vi "GetCtrlData.vi"(8 "error in (no error)":errorcluster, 11 "Panel in":refnum<vi>) -> (0 "error out":errorcluster, 2 "Indicators":string[][](array[string]), 3 "Controls":string[][](array[string]))   [LabVIEW 2016, in "update vi properties.lvlib"]
uses:
  update vi properties.lvlib
panel:
  # "Connector Pane"
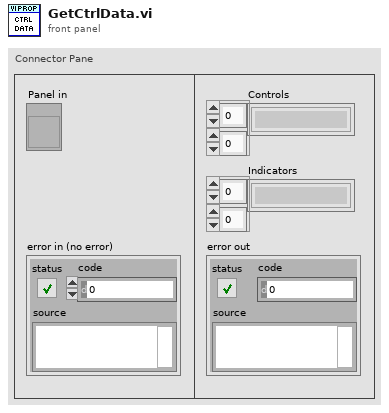
[diagram p1: front panel]
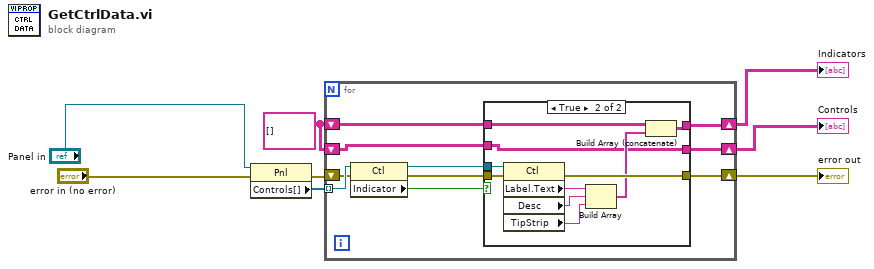
[diagram p0: block diagram]
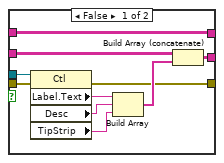
[diagram p2: hidden frame]
diagram:
  w8 = string[][] []
  n1 = property class="Pnl"(reference="Panel in", error in="error in (no error)") -> (error out=w7:errorcluster, "Controls[]"=w6:refnum<vi>[])  [unwired: 1 out]
  n2 = for {
    tunnel: w6 -> [w18] mode=indexing
    shift-right: [w13] -> w5
    shift-left: w7 -> [w17]
    shift-right: [w12] -> w3
    shift-left: w8 -> [w11]
    shift-right: [w10] -> w4
    shift-left: w8 -> [w9]
    n3 = property class="Ctl"(reference=w18, error in=w17) -> (reference out=w15:refnum<vi>, error out=w14:errorcluster, "Indicator"=w16:bool)
    n4 = case shown="True" w16 {
      tunnel: w15 -> [w23 w38]
      tunnel: w14 -> [w24 w37]
      tunnel: [w22 w36] -> w13
      tunnel: [w19 w30] -> w12
      tunnel: w11 -> [w19 w32]
      tunnel: [w21 w29] -> w10
      tunnel: w9 -> [w20 w29]
      frame False {
        n5 = property class="Ctl"(reference=w23, error in=w24) -> (error out=w22:errorcluster, "Label.Text"=w28:string, "Desc"=w27:string, "TipStrip"=w26:string)  [unwired: 1 out]
        n6 = Build Array(w28, w27, w26) -> (w25:string[])
        n7 = Build Array (concatenate)(w20, w25) -> (w21:string[][])
      }
      frame True {
        n8 = property class="Ctl"(reference=w38, error in=w37) -> (error out=w36:errorcluster, "Label.Text"=w35:string, "Desc"=w34:string, "TipStrip"=w33:string)  [unwired: 1 out]
        n9 = Build Array(w35, w34, w33) -> (w31:string[])
        n10 = Build Array (concatenate)(w32, w31) -> (w30:string[][])
      }
    }
  }
  "error out" <- w5
  "Controls" <- w4
  "Indicators" <- w3
